vi "CalculateVelAtPoints.vi"(5 "DistanceSlowAtEnd":dbl=12.0 format="%#_13g", 6 "Spacing":dbl=6.0, 7 "SlowSpeed":dbl=15.0 format="%#_13g", 8 "MaxVels":dbl[](array[numeric])=[inf, 2157065.6627048375, 861626.112790811, 578671.6913331844, 429961.8801252585, 308121.9449244763, 207918.27906416025, 136177.3173430706, 89569.91528184632, 58800.18152459611, 39880.76762584859, 26194.80445009087, 17829.217594495425, 11845.17306978302, 7879.569968013148, 5253.324793932985, 3469.547856398936, 2277.4904021580896, 1481.2285760407578, 948.0959476994294, 592.7427658361065, 357.4673686325199, 203.90457918870422, 106.75951370065539, 49.306559315345176, 20.128999935163755, 15.35216434544384, 33.658808151755416, 74.82922769308516, 162.02321338490634, 497.50383494931606, inf], 9 "MaxVel":dbl=100.0, 10 "MaxAccel":dbl=70.0, 11 "DistancesToEnd":dbl[](array[numeric])=[166.7705973927969, 160.77084408380804, 154.7711435600488, 148.77156499009723, 142.77217447548597, 136.77305100864692, 130.77431366598142, 124.77615392943866, 118.7788686907261, 112.78291387002021, 106.78894183411117, 100.79795865489717, 94.81140421691798, 88.83144545824503, 82.86133605354851, 76.90588123195663, 70.97226078269284, 65.07113856302844, 59.21840834916028, 53.43751144945011, 47.76306026298875, 42.245768335915066, 36.95893228065257, 32.00577775003234, 27.52281729491167, 23.656823188580333, 20.41267897914544, 16.87350007898272, 12.87686920812629, 8.580569476595137, 4.20703187879945, 0.0]) -> (3 "Vel":dbl[](array[numeric])=[100.0, 100.0, 100.0, 100.0, 100.0, 100.0, 100.0, 100.0, 100.0, 100.0, 100.0, 100.0, 100.0, 97.61979182595545, 93.24059437544017, 88.65689349657195, 83.84114682878314, 78.76027419208593, 73.37437264379857, 67.63485044643473, 61.482109827225365, 54.841854080771974, 47.61797886596968, 39.67405042333216, 30.763871883691905, 20.128999935163755, 15.35216434544384, 33.658808151755416, 37.93121703960681, 28.936054736114187, 15.0, 0.0])   [LabVIEW 2018]
doc: "Finds the target velocity at each point, taking in a list of maximum velocities based on curvature, and the max velocity and acceleration. \n\nWorks backwards through the path and limits the acceleration."
panel:
  out "Waveform Graph":dbl[](graph)=[100.0, 100.0, 100.0, 100.0, 100.0, 100.0, 100.0, 100.0, 100.0, 100.0, 100.0, 100.0, 100.0, 97.61979182595545, 93.24059437544017, 88.65689349657195, 83.84114682878314, 78.76027419208593, 73.37437264379857, 67.63485044643473, 61.482109827225365, 54.841854080771974, 47.61797886596968, 39.67405042333216, 30.763871883691905, 20.128999935163755, 15.35216434544384, 33.658808151755416, 37.93121703960681, 28.936054736114187, 15.0, 0.0]
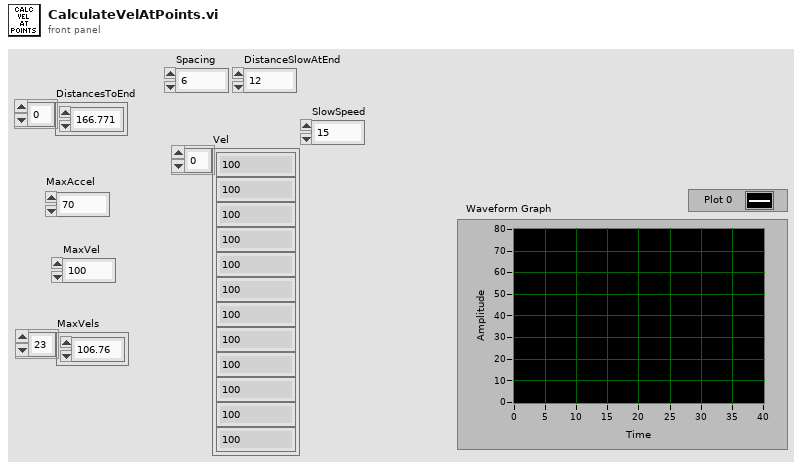
[diagram p1: front panel]
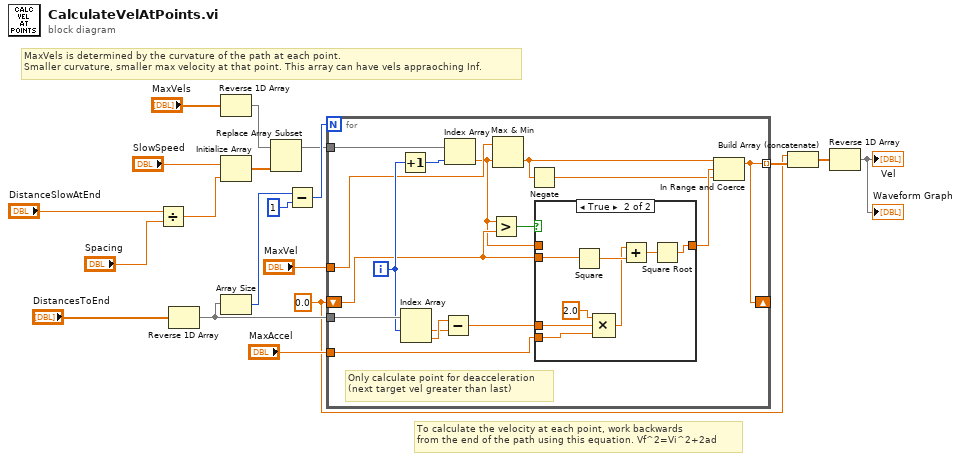
[diagram p0: block diagram]
diagram:
  w11 = 0.0 ("MaxAccel")
  # "MaxVels is determined by the curvature of the path at each point.\nSmaller curvature, smaller max velocity at that point. This array can have vels appraoching Inf."
  # "To calculate the velocity at each point, work backwards\nfrom the end of the path using this equation. Vf^2=Vi^2+2ad"
  n1 = Divide(x="DistanceSlowAtEnd", y="Spacing") -> (x/y=w1:dbl)
  n2 = Reverse 1D Array(array="DistancesToEnd") -> (reversed array=w13:dbl[])
  n3 = Reverse 1D Array(array="MaxVels") -> (reversed array=w2:dbl[])
  n4 = Initialize Array("SlowSpeed", w1) -> (w7:dbl[])
  n5 = Array Size(array=w13) -> (size(s)=w19:i32)
  n6 = Replace Array Subset(array=w2, new element=w7) -> (w8:dbl[])  [unwired: 1 in]
  n7 = Subtract(x=w19, y=1) -> (x-y=w17:i32)
  n8 = for {
    N: w17 -> [_]
    tunnel: w13 -> [w35]
    shift-right: [w24] -> _
    shift-left: w11 -> [w27]
    tunnel: "MaxAccel" -> [w26]
    tunnel: "MaxVel" -> [w22]
    tunnel: w8 -> [w32]
    tunnel: [w24] -> w12 mode=indexing
    i -> [w31]
    # "Only calculate point for deacceleration\n(next target vel greater than last)"
    n9 = Increment(x=w31) -> (x+1=w30:i32)
    n10 = Index Array(array=w35, index #1=w31) -> (element #1=w33:dbl, element #2=w34:dbl)  [unwired: 1 in]
    n11 = Subtract(x=w34, y=w33) -> (x-y=w28:dbl)
    n12 = Index Array(array=w32, index=w30) -> (element=w21:dbl)
    n13 = Greater?(x=w21, y=w27) -> (0:w29:bool)
    n14 = Max & Min(x=w22, y=w21) -> (min(x,y)=w20:dbl)  [unwired: 1 out]
    n15 = Negate(x=w20) -> (-x=w23:dbl)
    n16 = case shown="True" w29 {
      tunnel: w28 -> [_ w42]
      tunnel: [w36 w37] -> w25
      tunnel: w27 -> [_ w44]
      tunnel: w21 -> [w36 _]
      tunnel: w26 -> [_ w41]
      frame False {
      }
      frame True {
        n17 = Square(x=w44) -> (x^2=w40:dbl)
        n18 = Compound Arithmetic op=MULTIPLY(2.0 ("value"), w42, w41) -> (w39:dbl)
        n19 = Add(x=w39, y=w40) -> (x+y=w38:dbl)
        n20 = Square Root(x=w38) -> (sqrt(x)=w37:dbl)
      }
    }
    n21 = In Range and Coerce(upper limit=w20, x=w25, lower limit=w23) -> (coerced(x)=w24:dbl)  [unwired: 1 out]
  }
  n22 = Build Array (concatenate)(w11, w12) -> (w10:dbl[])
  n23 = Reverse 1D Array(array=w10) -> (reversed array=→"Vel" →"Waveform Graph":dbl[])
